vi "灰度分析.vi"() -> ()   [LabVIEW 2018]
uses:
  <vilib>/vision/NI_Vision_Development_Module.lvlib
panel:
  out "error out":errorcluster
  out "波形图":sgl[](graph)
  out "Image":T1(plugin-control)
  in  "路径":path
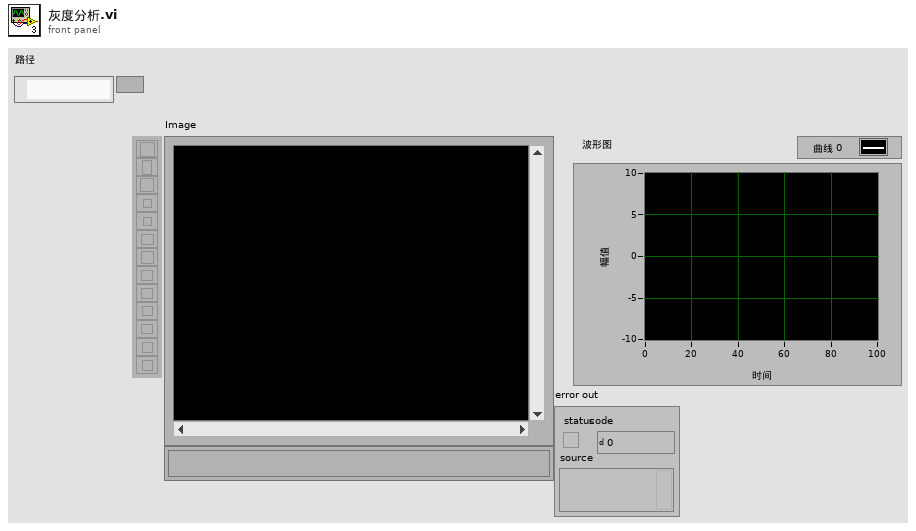
[diagram p1: front panel]
types:
  T1 = typedef "IMAQ Image.ctl" = refnum<image>
  T2 = cluster{"Left":i32, "Top":i32, "Right":i32, "Bottom":i32}
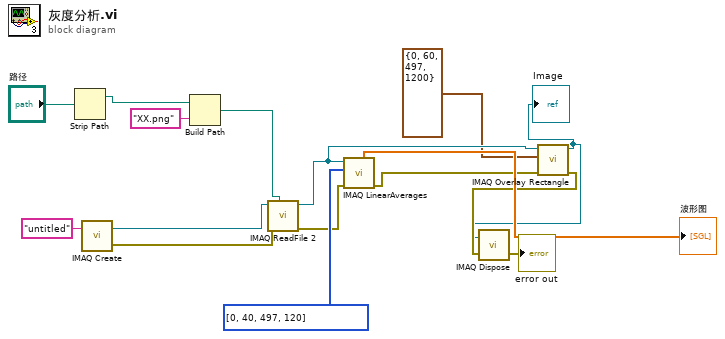
[diagram p0: block diagram]
diagram:
  n1 = Strip Path(path="路径") -> (stripped path=w15:path)  [unwired: 1 out]
  n2 = call "IMAQ Create"("Image Name"="untitled") -> ("New Image"=w13:T1, "error out"=w12:errorcluster)  [unwired: 4 in]
  n3 = Build Path(base path=w15, name or relative path="XX.png" ("名称或相对路径")) -> (appended path=w10:path)
  n4 = call "IMAQ ReadFile 2"("File Path"=w10, "error in (no error)"=w12, "Image"=w13) -> ("error out"=w8:errorcluster, "Image Out"=w6:T1)  [unwired: 4 in, 3 out]
  n5 = call "IMAQ LinearAverages"("error in (no error)"=w8, "Optional Rectangle"=i32[] [0, 40, 497, 120], "Image Src"=w6) -> ("error out"=w5:errorcluster, "X Axis Averages"=→"波形图":sgl[])  [unwired: 4 in, 3 out]
  n6 = call "IMAQ Overlay Rectangle"("error in (no error)"=w5, "Rectangle"=T2 {"Left"=0, "Top"=60, "Right"=497, "Bottom"=1200}, "Image"=w6) -> ("error out"=w4:errorcluster, "Image Out"=w3:T1)  [unwired: 7 in]
  "Image" <- w3
  n7 = call "IMAQ Dispose"("Image"=w3, "error in (no error)"=w4) -> ("error out"=→"error out":errorcluster)  [unwired: 4 in]
